vi "CloseXL_Worksheet.vi"(8 "error in (no error)":errorcluster, 11 "Refnum Cluster In":T1) -> (0 "error out":errorcluster, 3 "Refnum Cluster Out":T2)   [LabVIEW 2015]
doc: "This VI closes the previously opened Excel spreadsheet. The workbook remains open, though, which allows another spreadsheet to be opened."
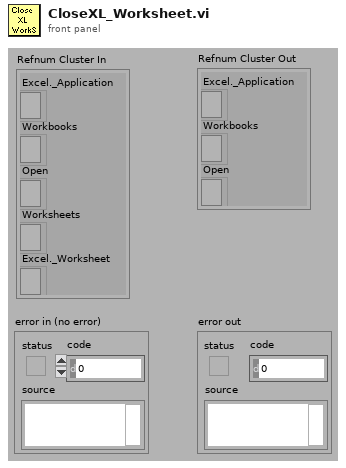
[diagram p1: front panel]
types:
  T1 = cluster{"Excel._Application":refnum<k7>, "Workbooks":refnum<k7>, "Open":refnum<k7>, "Worksheets":refnum<k7>, "Excel._Worksheet":refnum<k7>}
  T2 = cluster{"Excel._Application":refnum<k7>, "Workbooks":refnum<k7>, "Open":refnum<k7>}
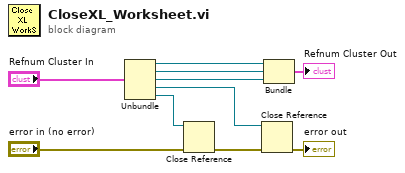
[diagram p0: block diagram]
diagram:
  n1 = Unbundle("Refnum Cluster In") -> ("Excel._Application"=w7:refnum<k7>, "Workbooks"=w8:refnum<k7>, "Open"=w9:refnum<k7>, "Worksheets"=w3:refnum<k7>, "Excel._Worksheet"=w4:refnum<k7>)
  n2 = Close Reference(reference=w4, error in (no error)="error in (no error)") -> (error out=w2:errorcluster)
  n3 = Close Reference(reference=w3, error in (no error)=w2) -> (error out=→"error out":errorcluster)
  n4 = Bundle("Excel._Application"=w7, "Workbooks"=w8, "Open"=w9) -> (→"Refnum Cluster Out":T2)  [unwired: 1 in]
